vi "Create Server.vi"(8 "error in":errorcluster) -> (0 "error out":errorcluster, 3 "gRPCid out":T1)   [LabVIEW 2019, in "grpc-lvsupport.lvlib"]
uses:
  grpc-lvsupport.lvlib
  Shared/grpcId.ctl
  <vilib>/Utility/error.llb/Error Cluster From Error Code.vi
  <resource>/labview_grpc_server.dll
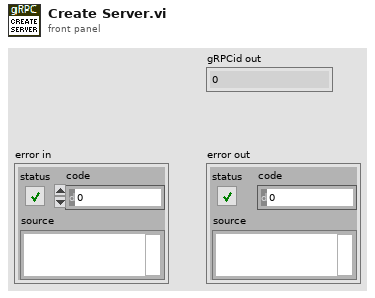
[diagram p1: front panel]
types:
  T1 = typedef "grpc-lvsupport.lvlib/grpcId.ctl" = u64
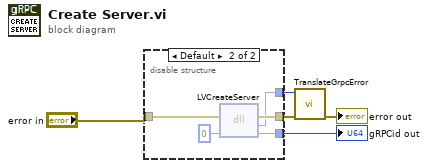
[diagram p0: block diagram]
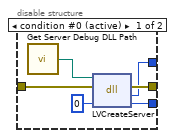
[diagram p2: hidden frame]
diagram:
  n1 = disable-structure shown="Default" {
    disable-tunnel: "error in" -> [w11 w16]
    disable-tunnel: [w10 w15] -> w4
    disable-tunnel: [w9 w14] -> w3
    disable-tunnel: [w7 w13] -> w1
    frame condition #0 (active) {
      n2 = call "Get Server Debug DLL Path.vi"() -> ("Server Debug DLL Path"=w8:path)
      n3 = dll-call lib="C:/Users/XEnderMD/Desktop/LV gRPC/labview source/gRPC interface/dlls/labview_grpc_server.dll" fn="LVCreateServer"(path in=w8, error in=w11, "gRPCid out"=T1 0) -> (error out=w10:errorcluster, "return type"=w7:i32, "gRPCid out"=w9:T1)  [unwired: 1 in, 1 out]
    }
    frame condition #1 {
      n4 = dll-call lib="C:/Program Files (x86)/National Instruments/LabVIEW 2024/resource/labview_grpc_server.*" fn="LVCreateServer"(error in=w16, "server"=T1 0 ("gRPCid out")) -> (error out=w15:errorcluster, "return type"=w13:i32, "server"=w14:T1)  [unwired: 2 in, 1 out]
    }
  }
  "gRPCid out" <- w3
  n5 = call "TranslateGrpcError.vi"("error in"=w4, "Error Code"=w1) -> ("error out"=→"error out":errorcluster)  [unwired: 9 in]
